vi "Test Object Datatype.vi"(8 "error in (no error)":errorcluster) -> (0 "error out":errorcluster)   [LabVIEW 2018, in "JSON to LVConstant Test.lvlib"]
uses:
  JSON to LVConstant Test.lvlib
  <vilib>/JDP Science/JSONtext/JSON Value Type.ctl
  <vilib>/addons/_JKI Toolkits/Caraya/classes/Test/Test.lvclass
  <vilib>/JDP Science/JSONtext/JSONtext.lvlib
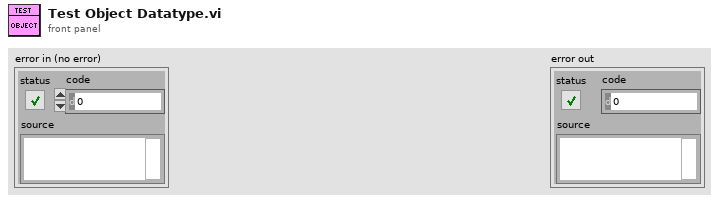
[diagram p1: front panel]
types:
  T1 = typedef "JSONtext.lvlib/JSON Value Type.ctl" = enum16{"Not a JSON Value", "JSON Object", "JSON Array", "String", "Number", "true", "false", "null"}
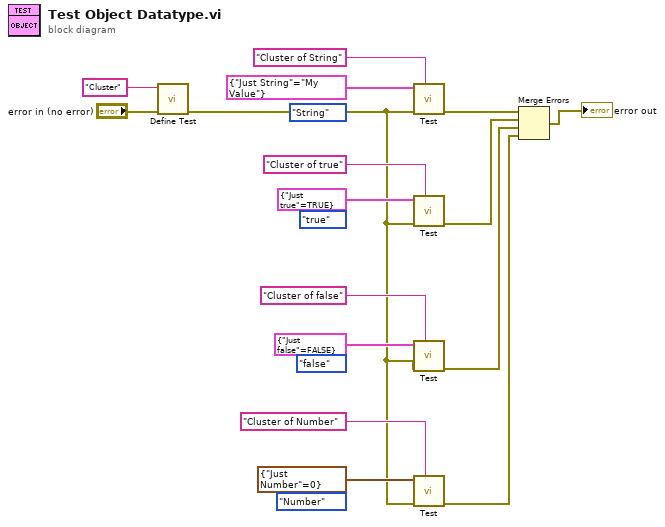
[diagram p0: block diagram]
diagram:
  (unwired) JSON_Value_Type."Number" ("JSON Value Type")
  (unwired) JSON_Value_Type."false" ("JSON Value Type")
  (unwired) JSON_Value_Type."true" ("JSON Value Type")
  (unwired) JSON_Value_Type."String" ("JSON Value Type")
  n1 = call <vilib>:"Define Test.vi"("error in (no error)"="error in (no error)", "Label (VI Title)"="Cluster") -> ("error out"=w2:errorcluster)  [unwired: 9 in]
  n2 = call "Test.vi"("Label (VI Title)"="Cluster of String", "error in (no error)"=w2, "Type"=cluster{"Just String":string} {"Just String"="My Value"}) -> ("error out"=w13:errorcluster)  [unwired: 8 in]
  n3 = call "Test.vi"("Label (VI Title)"="Cluster of true", "error in (no error)"=w2, "Type"=cluster{"Just true":bool} {"Just true"=TRUE}) -> ("error out"=w9:errorcluster)  [unwired: 8 in]
  n4 = call "Test.vi"("Label (VI Title)"="Cluster of false", "error in (no error)"=w2, "Type"=cluster{"Just false":bool} {"Just false"=FALSE}) -> ("error out"=w10:errorcluster)  [unwired: 8 in]
  n5 = call "Test.vi"("Label (VI Title)"="Cluster of Number", "error in (no error)"=w2, "Type"=cluster{"Just Number":i32} {"Just Number"=0}) -> ("error out"=w11:errorcluster)  [unwired: 8 in]
  n6 = Merge Errors(w13, w9, w10, w11) -> (→"error out":errorcluster)
